vi "config_optom.vi"() -> ()   [LabVIEW 2017]
panel:
  in  "System Tab":T1(tab)
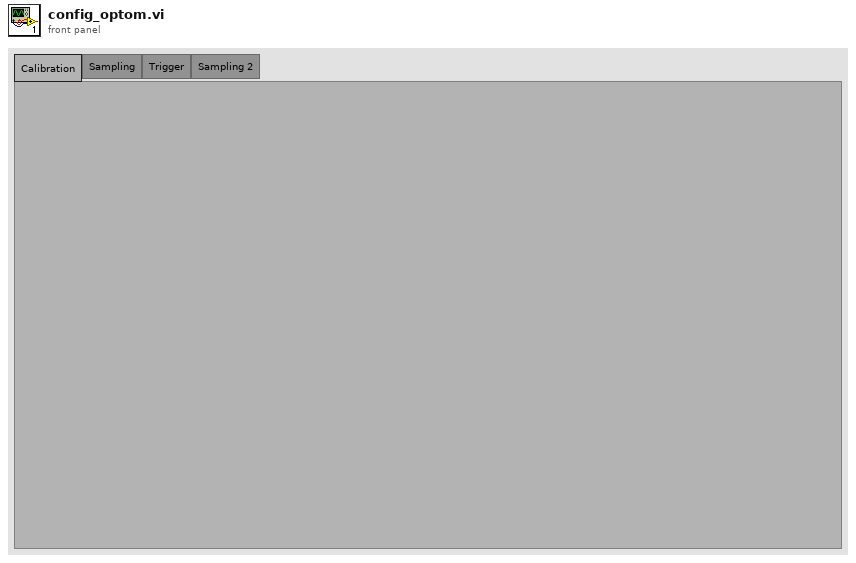
[diagram p1: front panel]
types:
  T1 = enum32{"Calibration", "Sampling", "Trigger", "Sampling 2"}
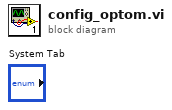
[diagram p0: block diagram]
diagram:
